vi "作业.vi"() -> ()   [LabVIEW 2018]
panel:
  in  "n":dbl
  in  "m":dbl
  in  "停止":bool
  in  "字符串 4":string
  out "反转的数组":i32[](array[numeric])
  out "数组 3":i32[](array[numeric])
  out "数组":i32[](array[numeric])
  out "转置的数组":dbl[][](array[numeric])
  out "y2":dbl
  out "y1":dbl
  in  "b":dbl
  in  "m":dbl
  out "字符串 3":string
  out "数组 2":dbl[][](array[numeric])=[[1.0, 2.0, 3.0], [4.0, 5.0, 6.0]] format="%.2g"
  out "x+y 2":dbl
  out "滑动杆 2":u8(slide) scale=0.0..100.0
  in  "字符串 2":string
  out "最小值":dbl
  out "x/y":dbl
  out "已删除元素的数组子集":i32[][](array[numeric])
  out "字符串":string
  out "输出变量":dbl
  in  "数值":dbl
  out "x+y":dbl
  # "1.(1)"
  # "1.(2)"
  # "2."
  # "3."
  # "4."
  # "5."
  # "6."
  # "7."
  # "8."
  # "9."
  # "10."
  # "11."
  # "12."
  # "13."
  # "14."
  # "15."
  # "16."
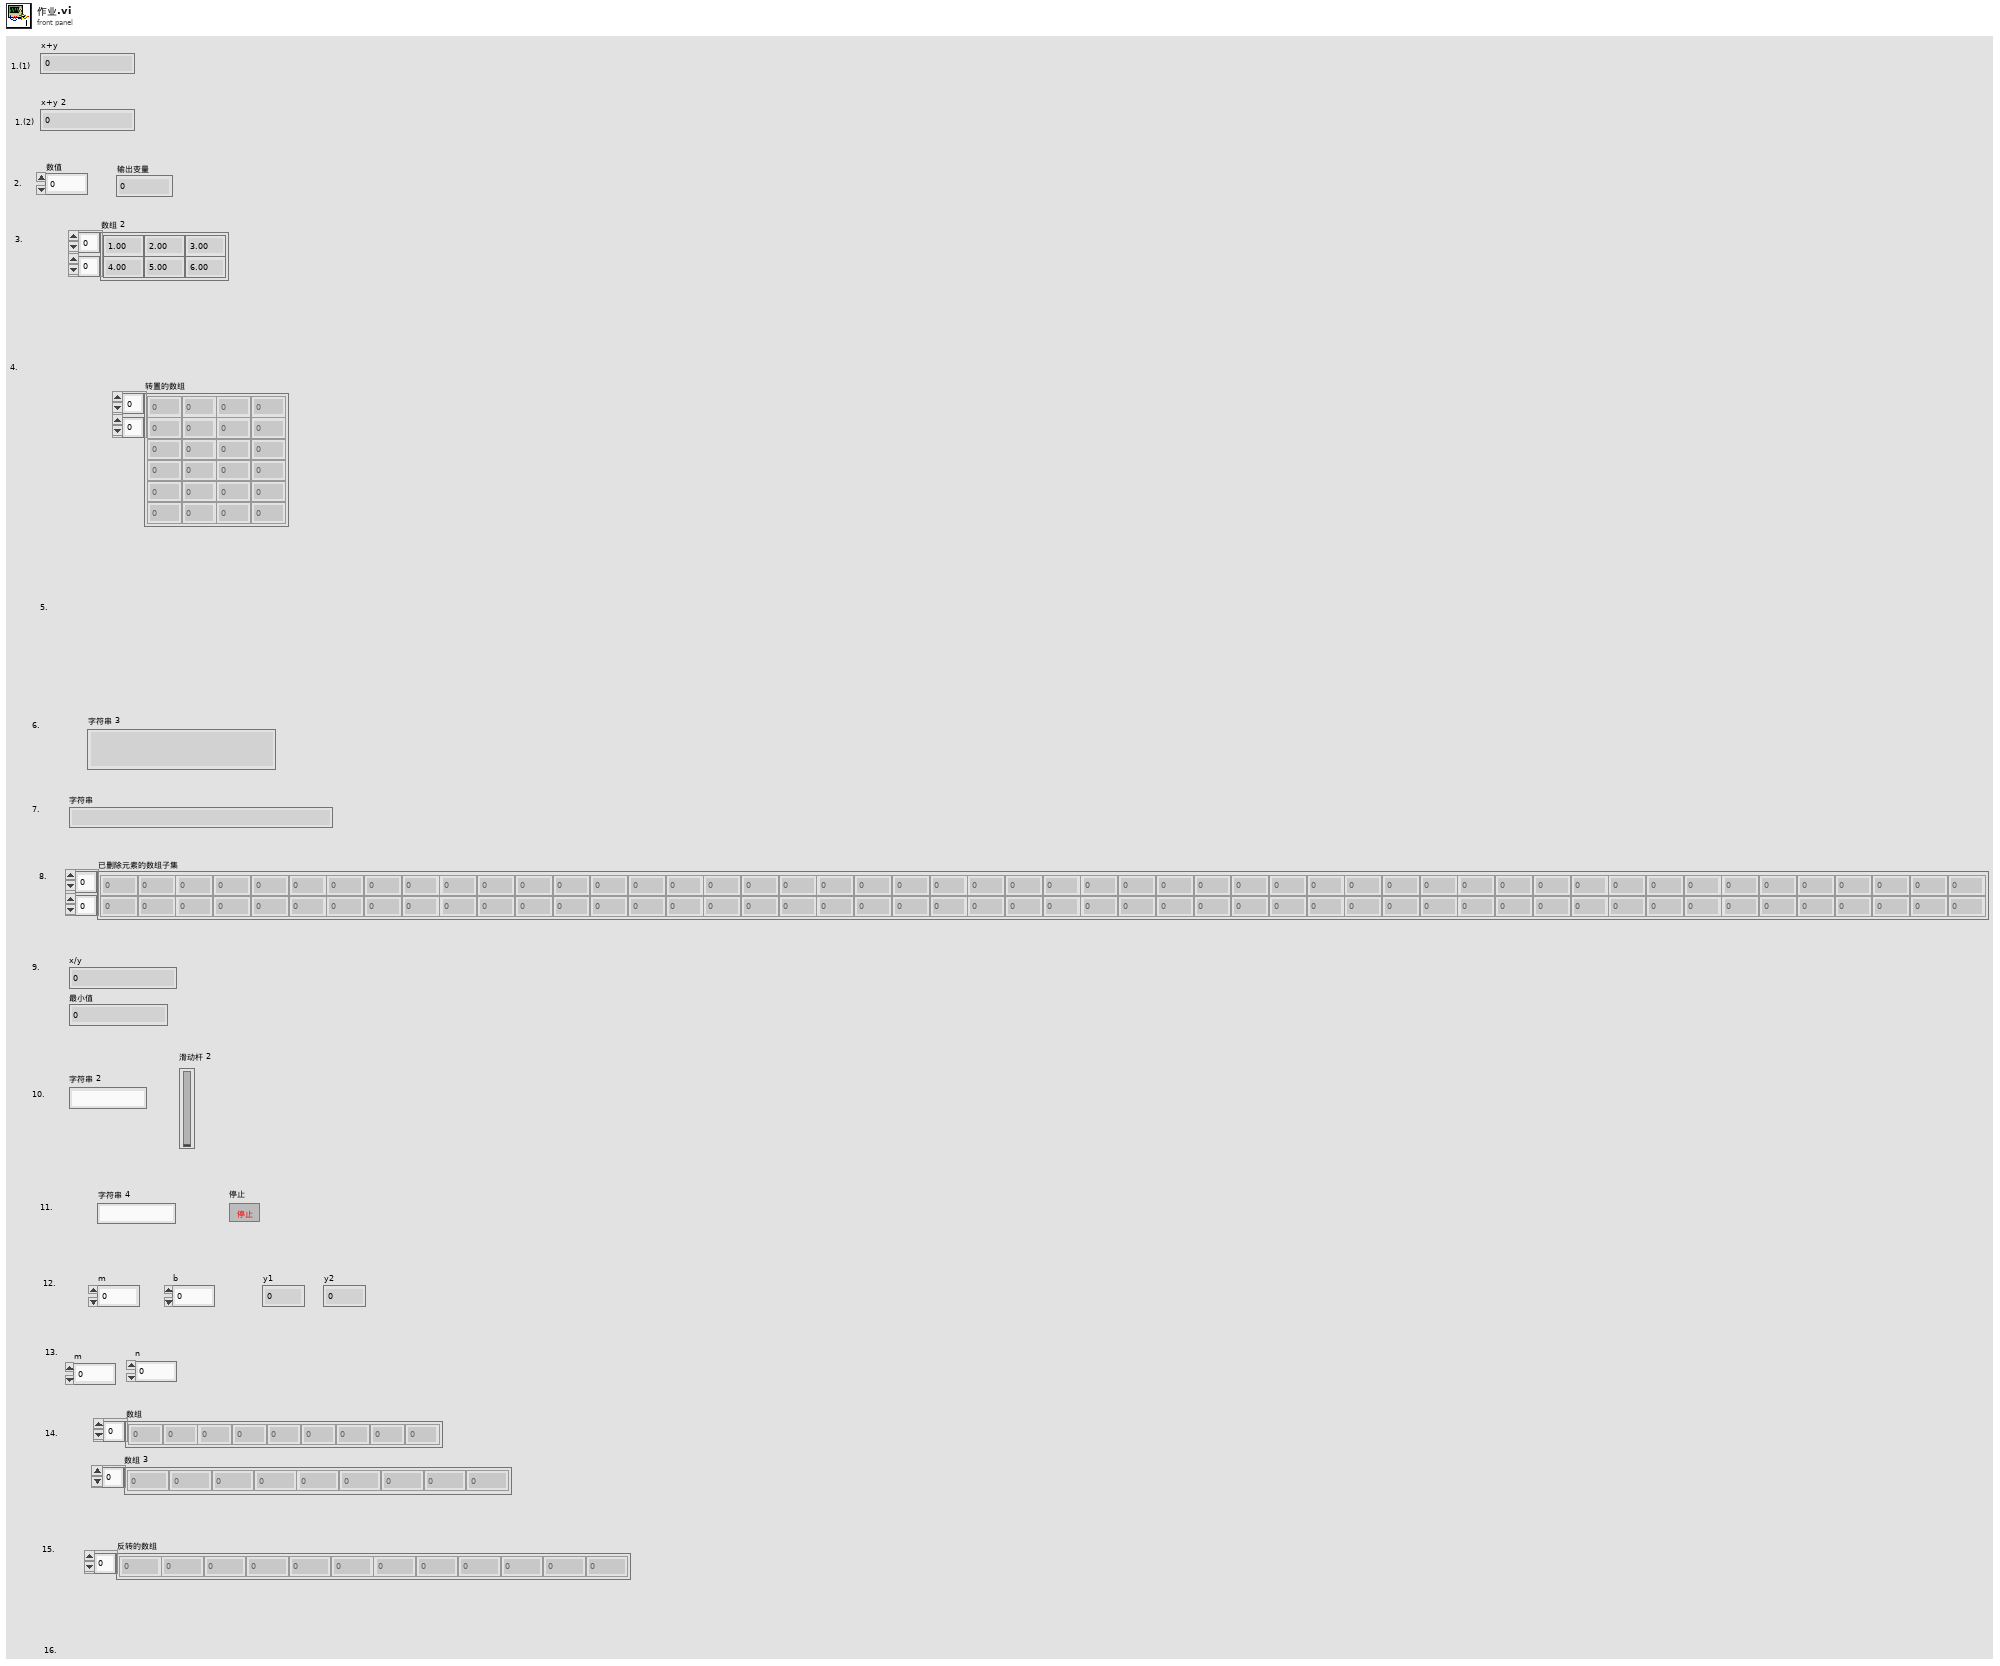
[diagram p1: front panel]
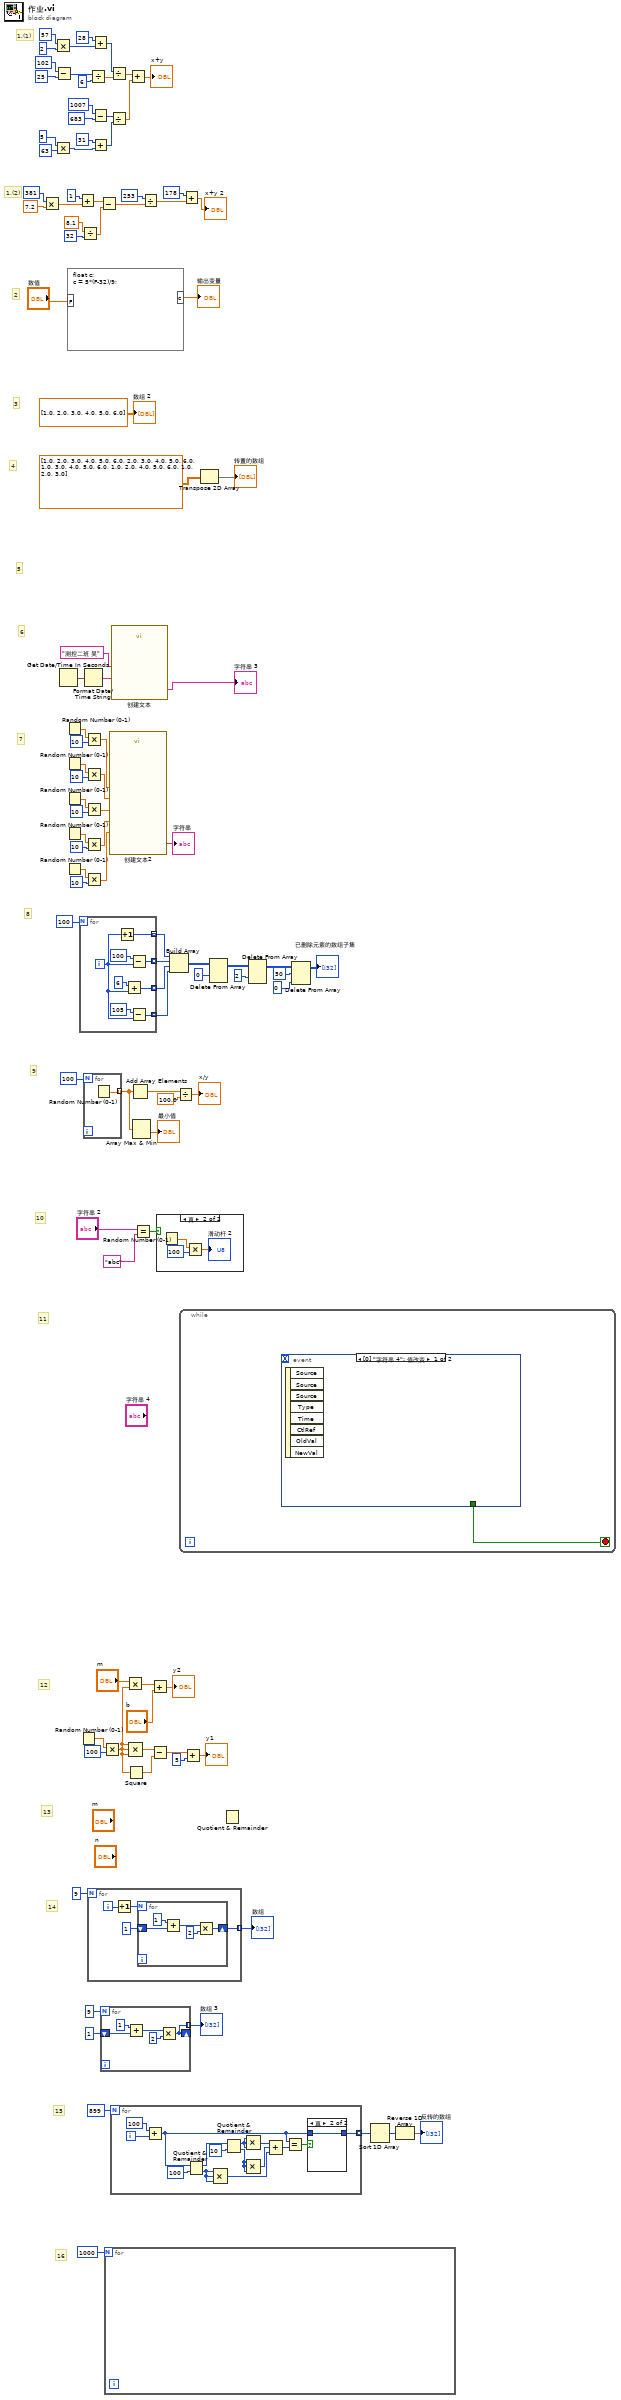
[diagram p0: block diagram]
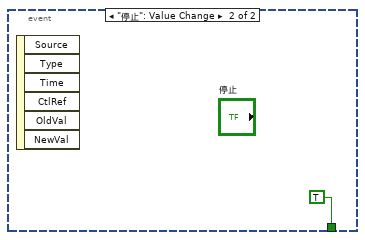
[diagram p2: hidden frame]
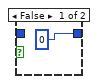
[diagram p3: hidden frame]
diagram:
  # "16"
  # "15"
  # "14"
  # "13"
  # "12"
  # "11"
  # "10"
  # "9"
  # "8"
  # "7"
  # "6"
  # "5"
  # "4"
  # "3"
  # "2"
  # "1.(2)"
  # "1.(1)"
  n1 = Multiply(x=381, y=7.2) -> (x*y=w35:dbl)
  n2 = Multiply(x=57, y=2) -> (x*y=w101:i32)
  n3 = Multiply(x=5, y=63) -> (x*y=w87:i32)
  n4 = Subtract(x=102, y=25) -> (x-y=w96:i32)
  n5 = Get Date/Time In Seconds() -> (seconds since 1Jan1904=w80:timestamp)
  n6 = Random Number (0-1)() -> (number: 0 to 1=w68:dbl)
  n7 = Random Number (0-1)() -> (number: 0 to 1=w70:dbl)
  n8 = Random Number (0-1)() -> (number: 0 to 1=w71:dbl)
  n9 = Random Number (0-1) ("随机数(0-10)")() -> (number: 0 to 1=w72:dbl)
  n10 = Random Number (0-1)() -> (number: 0 to 1=w69:dbl)
  n11 = formula code="float c;\nc = 5*(F-32)/9;"("F"="数值") -> ("c"=→"输出变量":dbl)
  n12 = Add(x=1, y=w35) -> (x+y=w32:dbl)
  n13 = for {
    N: 100 -> [_]
    tunnel: [w111] -> w60 mode=indexing
    tunnel: [w109] -> w57 mode=indexing
    tunnel: [w108] -> w58 mode=indexing
    tunnel: [w107] -> w59 mode=indexing
    i -> [w110]
    n14 = Increment(x=w110) -> (x+1=w111:i32)
    n15 = Add(x=6, y=w110) -> (x+y=w108:i32)
    n16 = Subtract(x=100, y=w110) -> (x-y=w107:i32)
    n17 = Subtract(x=105, y=w110) -> (x-y=w109:i32)
  }
  n18 = Random Number (0-1)() -> (number: 0 to 1=w24:dbl)
  n19 = Divide(x=8.1, y=32) -> (x/y=w31:dbl)
  n20 = for {
    N: 100 -> [_]
    tunnel: [w112] -> w47 mode=indexing
    n21 = Random Number (0-1)() -> (number: 0 to 1=w112:dbl)
  }
  n22 = Format Date/Time String(seconds (now)=w80) -> (date/time string=w79:string)  [unwired: 2 in]
  n23 = Multiply(x=w68, y=10) -> (x*y=w67:dbl)
  n24 = Multiply(x=w70, y=10) -> (x*y=w66:dbl)
  n25 = Multiply(x=w71, y=10) -> (x*y=w65:dbl)
  n26 = Multiply(x=w72, y=10) -> (x*y=w64:dbl)
  n27 = Multiply(x=w69, y=10) -> (x*y=w63:dbl)
  n28 = for {
    N: 9 -> [_]
    tunnel: [w113] -> w9 mode=indexing
    i -> [w115]
    n29 = Increment(x=w115) -> (x+1=w114:i32)
    n30 = for {
      N: w114 -> [_]
      shift-right: [w117] -> w113
      shift-left: 1 -> [w120]
      n31 = Add(x=1, y=w120) -> (x+y=w119:i32)
      n32 = Multiply(x=w119, y=2) -> (x*y=w117:i32)
    }
  }
  "数组" <- w9
  n33 = Divide(x=w96, y=6) -> (x/y=w94:dbl)
  n34 = Add(x=28, y=w101) -> (x+y=w95:i32)
  n35 = Subtract(x=1007, y=683) -> (x-y=w86:i32)
  n36 = Add(x=31, y=w87) -> (x+y=w85:i32)
  n37 = Subtract(x=w32, y=w31) -> (x-y=w29:dbl)
  n38 = for {
    N: 9 -> [_]
    shift-right: [w122] -> _
    shift-left: 1 -> [w125]
    tunnel: [w122] -> w6 mode=indexing
    n39 = Add(x=1, y=w125) -> (x+y=w124:i32)
    n40 = Multiply(x=w124, y=2) -> (x*y=w122:i32)
  }
  "数组 3" <- w6
  n41 = Multiply(x=w24, y=100) -> (x*y=w16:dbl)
  n42 = for {
    N: 1000 -> [_]
  }
  n43 = Divide(x=w95, y=w94) -> (x/y=w93:dbl)
  n44 = Divide(x=w86, y=w85) -> (x/y=w84:dbl)
  n45 = call "创建文本2"("4"=w64, "1"=w67, "2"=w66, "3"=w65, "5"=w63) -> ("Result"=→"字符串":string)  [unwired: 9 in, 1 out]
  n46 = for {
    N: 899 -> [_]
    tunnel: [w127] -> w4 mode=indexing
    i -> [w131]
    n47 = Add(x=100, y=w131) -> (x+y=w128:i32)
    n48 = Quotient & Remainder(x=w128, y=100) -> (x-y*floor(x/y)=w140:i32, floor(x/y)=w138:i32)
    n49 = Compound Arithmetic op=MULTIPLY(w138, w138, w138) -> (w133:i32)
    n50 = Quotient & Remainder(x=w140, y=10) -> (x-y*floor(x/y)=w136:i32, floor(x/y)=w137:i32)
    n51 = Compound Arithmetic op=MULTIPLY(w136, w136, w136) -> (w135:i32)
    n52 = Compound Arithmetic op=MULTIPLY(w137, w137, w137) -> (w134:i32)
    n53 = Compound Arithmetic op=ADD(w135, w134, w133) -> (w132:i32)
    n54 = Equal?(x=w128, y=w132) -> (x = y?=w129:bool)
    n55 = case shown="真" w129 {
      tunnel: w128 -> [_ w143]
      tunnel: [0 w143] -> w127
      frame False {
      }
      frame True {
      }
    }
  }
  n56 = call "创建文本"("a"="测控二班 吴", "b"=w79) -> ("Result"=→"字符串 3":string)  [unwired: 12 in, 1 out]
  n57 = Multiply(x="m", y=w16) -> (x*y=w15:dbl)
  n58 = Square(x=w16) -> (x^2=w21:dbl)
  n59 = Compound Arithmetic op=MULTIPLY(w16, w16, w16) -> (w22:dbl)
  n60 = Add(x=w93, y=w84) -> (x+y=→"x+y":dbl)
  n61 = Add Array Elements(numeric array=w47) -> (sum=w46:dbl)
  n62 = Array Max & Min(array=w47) -> (min value=→"最小值":dbl)  [unwired: 3 out]
  n63 = Equal?(x="字符串 2", y="abc") -> (x = y?=w40:bool)
  n64 = Divide(x=253, y=w29) -> (x/y=w28:dbl)
  n65 = Add(x=w15, y="b") -> (x+y=→"y2":dbl)
  n66 = Subtract(x=w22, y=w21) -> (x-y=w20:dbl)
  n67 = case shown="真" w40 {
    frame False {
    }
    frame True {
      n68 = Random Number (0-1)() -> (number: 0 to 1=w146:dbl)
      n69 = Multiply(x=w146, y=100) -> (x*y=→"滑动杆 2":dbl)
    }
  }
  n70 = Build Array(w60, w59, w58, w57) -> (w56:i32[][])
  n71 = Divide(x=w46, y=100.0) -> (x/y=→"x/y":dbl)
  n72 = while {
    stop <- w147 stop-if-true
    n73 = event shown="[0] \"字符串 4\": 值改变" {
      selector: _ -> [_ _]
      dyn-events: _ -> [_ _]
      timeout: _ -> [_ _]
      tunnel: [_ TRUE] -> w147
      event "字符串 4": Value Change {
        n74 = event-data() -> ()  [unwired: 1 in, 8 out]
      }
      event "停止": Value Change {
        n75 = event-data() -> ()  [unwired: 1 in, 6 out]
      }
    }
  }
  n76 = Add(x=178, y=w28) -> (x+y=→"x+y 2":dbl)
  n77 = Add(x=w20, y=5) -> (x+y=→"y1":dbl)
  n78 = Transpose 2D Array(2D array=dbl[][] [[1.0, 2.0, 3.0, 4.0, 5.0, 6.0], [2.0, 3.0, 4.0, 5.0, 6.0, 1.0], [3.0, 4.0, 5.0, 6.0, 1.0, 2.0], [4.0, 5.0, 6.0, 1.0, 2.0, 3.0]]) -> (transposed array=→"转置的数组":dbl[][])
  n79 = Delete From Array(array=w56, index (row)=0 ("索引 (行)")) -> (array with subset deleted=w54:i32[][])  [unwired: 2 in, 1 out]
  n80 = Quotient & Remainder() -> ()  [unwired: 2 in, 2 out]
  n81 = Delete From Array(array=w54, index (row)=2 ("索引 (行)")) -> (array with subset deleted=w52:i32[][])  [unwired: 2 in, 1 out]
  n82 = Delete From Array(array=w52, length=50, index (col)=0) -> (array with subset deleted=→"已删除元素的数组子集":i32[][])  [unwired: 1 in, 1 out]
  n83 = Sort 1D Array(array=w4) -> (sorted array=w3:i32[])
  n84 = Reverse 1D Array(array=w3) -> (reversed array=→"反转的数组":i32[])
  "数组 2" <- dbl[][] [[1.0, 2.0, 3.0], [4.0, 5.0, 6.0]]
